vi "dI-dV and Delta.vi"(5 "V offset":dbl, 6 "I offset":dbl, 7 "How many V sweep periods?":dbl=1.0, 8 "Input data":cluster{dbl[], dbl[]}(graph), 9 "dI/dV (Delta) Parameters":T1={"High voltage value"=0.0005, "Low voltage value"=-0.0005, "decimation points"=600, "side points"=4, "polynomial order 2"=3, "valley width"=10, "valley threshold"=1.3e-05, "conductance-peak threshold"=2e-05}) -> (0 "Delta (V)":dbl=7.833333333333333e-05, 1 "Delta":cluster{"2*Delta (V)":dbl, "Delta (V)":dbl}={"2*Delta (V)"=0.00015666666666666666, "Delta (V)"=7.833333333333333e-05} {"2*Delta (V)" format="%#_6p"; "Delta (V)" format="%#_6p"}, 2 "dI/dV and Delta valleys":cluster{"X Subset":dbl[], "Filtered X":dbl[]}[](graph), 3 "I vs V - Offset Plot":cluster{dbl[], dbl[]}[](graph), 4 "Data for second derivative":cluster{"xi used":dbl[], "dX/dt":dbl[]})   [LabVIEW 2016]
uses:
  <vilib>/Analysis/3filter.llb/Savitzky-Golay Filter (DBL).vi
  <vilib>/Analysis/NI_AALPro.lvlib
  <vilib>/gmath/NI_Gmath.lvlib
  <vilib>/Analysis/NI_AALBase.lvlib
  <vilib>/Analysis/NI_AAL_SigProc.lvlib
panel:
  out "High voltage value":dbl=0.0005
  out "Low voltage value":dbl=-0.0005
  out "decimation points":i32=600
  out "side points":i32=4
  out "polynomial order 2":i32=3
  out "valley width":i32=10
  out "valley threshold":dbl=1.3e-05
  out "conductance-peak threshold":dbl=2e-05
  # "paste data here"
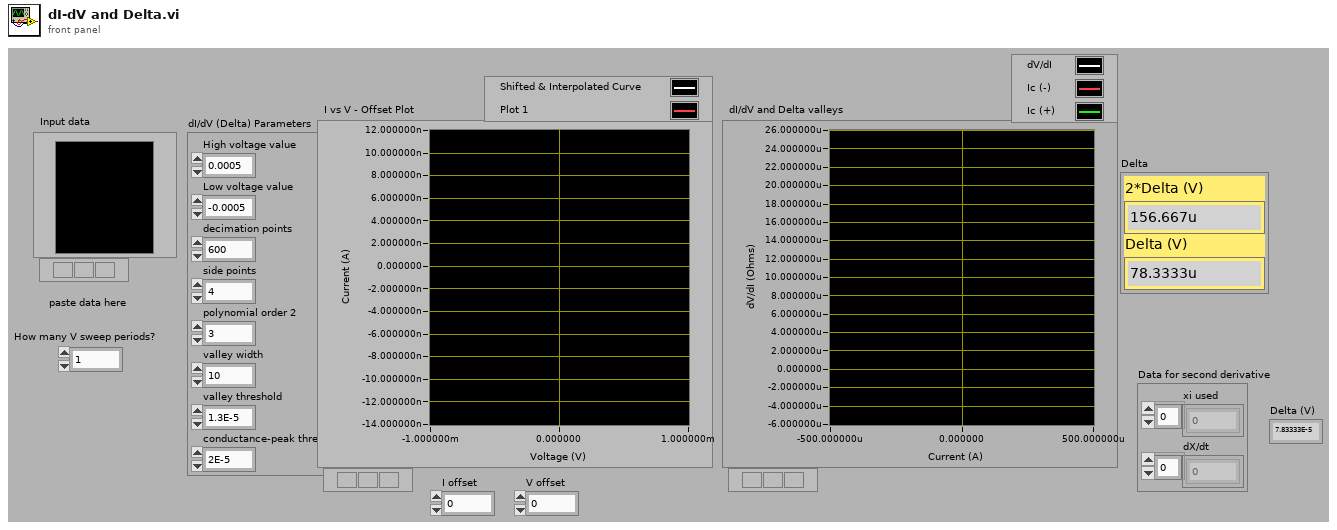
[diagram p1: front panel]
types:
  T1 = cluster{"High voltage value":dbl, "Low voltage value":dbl, "decimation points":i32, "side points":i32, "polynomial order 2":i32, "valley width":i32, "valley threshold":dbl, "conductance-peak threshold":dbl}
  T2 = cluster{"Positive Val":dbl, "Negative Val":dbl, "Ave Ic":dbl}
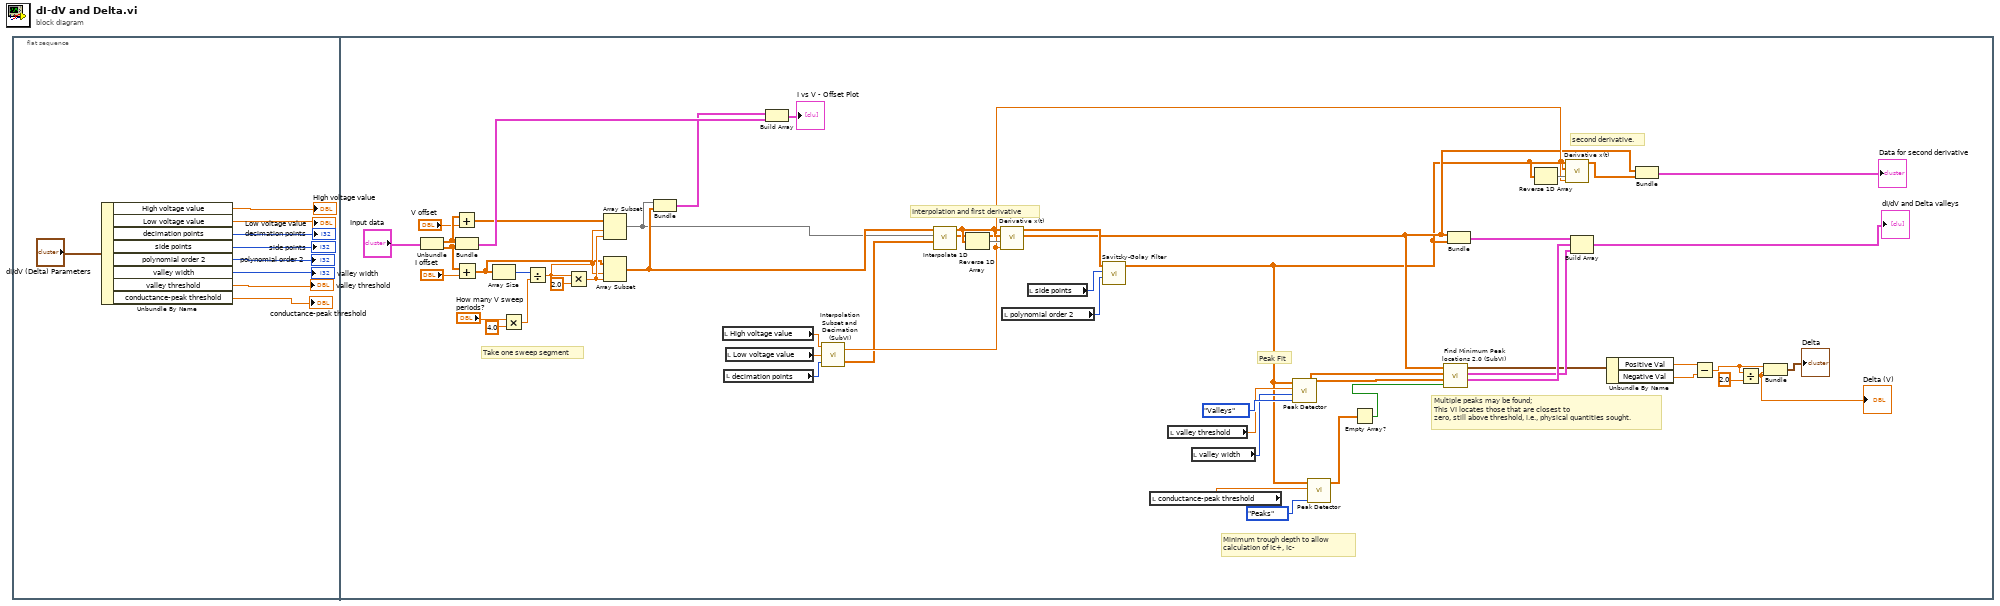
[diagram p0: block diagram]
diagram:
  n1 = flat-sequence {
    frame #0 {
      n2 = Unbundle By Name("dI/dV (Delta) Parameters") -> ("High voltage value"=→"High voltage value":dbl, "Low voltage value"=→"Low voltage value":dbl, "decimation points"=→"decimation points":i32, "side points"=→"side points":i32, "polynomial order 2"=→"polynomial order 2":i32, "valley width"=→"valley width":i32, "valley threshold"=→"valley threshold":dbl, "conductance-peak threshold"=→"conductance-peak threshold":dbl)
    }
    frame #1 {
      # "second derivative."
      # "Multiple peaks may be found;\nThis VI locates those that are closest to\nzero, still above threshold, i.e., physical quantities sought."
      # "Minimum trough depth to allow \ncalculation of Ic+, Ic-"
      # "Peak Fit"
      # "Interpolation and first derivative"
      # "Take one sweep segment"
      n3 = Unbundle("Input data") -> (w61:dbl[], w62:dbl[])
      n4 = Add(x=w61, y="V offset") -> (x+y=w50:dbl[])
      n5 = Bundle(w61, w62) -> (w63:cluster{dbl[], dbl[]})  [unwired: 1 in]
      n6 = Add(x=w62, y="I offset") -> (x+y=w55:dbl[])
      n7 = Array Size(array=w55) -> (size(s)=w51:i32)
      n8 = Multiply(x="How many V sweep periods?", y=4.0) -> (x*y=w52:dbl)
      n9 = Divide(x=w51, y=w52) -> (x/y=w56:dbl)
      n10 = Multiply(x=w56, y=2.0) -> (x*y=w57:dbl)
      n11 = Array Subset(array=w50, index=w56, length=w57) -> (w58:dbl[])
      n12 = Array Subset(array=w55, index=w56, length=w57) -> (w59:dbl[])
      n13 = Bundle(w58, w59) -> (w60:cluster{dbl[], dbl[]})  [unwired: 1 in]
      n14 = local read "High voltage value"() -> (w23:dbl)
      n15 = local read "decimation points"() -> (w21:i32)
      n16 = local read "Low voltage value"() -> (w22:dbl)
      n17 = Build Array(w60, w63) -> (→"I vs V - Offset Plot":cluster{dbl[], dbl[]}[])
      n18 = call "Interpolation Subset and Decimation (SubVI).vi"("decimation points"=w21, "Low value"=w22, "High value"=w23) -> ("Points to use in interpolation (xi)"=w34:dbl[], "Numeric"=w35:dbl)
      n19 = call <vilib>:"Interpolate 1D.vi"("xi"=w34, "X"=w58, "Y"=w59) -> ("xi used"=w29:dbl[], "yi"=w45:dbl[])  [unwired: 6 in, 1 out]
      n20 = Reverse 1D Array(array=w45) -> (reversed array=w46:dbl[])
      n21 = call <vilib>:"Derivative x(t).vi"("dt"=w35, "Final Condition"=w46, "Initial Condition"=w45, "X"=w45) -> ("dX/dt"=w44:dbl[])  [unwired: 6 in, 1 out]
      n22 = local read "polynomial order 2"() -> (w25:i32)
      n23 = local read "side points"() -> (w24:i32)
      n24 = call-poly <vilib>:"Savitzky-Golay Filter.vi"("polynomial order"=w25, "side points"=w24, "X"=w44) -> ("Filtered X"=w19:dbl[])  [unwired: 7 in, 1 out]
      n25 = local read "conductance-peak threshold"() -> (w28:dbl)
      n26 = local read "valley threshold"() -> (w27:dbl)
      n27 = local read "valley width"() -> (w26:i32)
      n28 = call <vilib>:"Peak Detector.vi"("peaks/valleys"=enum32{"Peaks", "Valleys"}."Valleys", "width"=w26, "threshold"=w27, "X"=w19) -> ("Amplitudes"=w37:dbl[], "Locations"=w36:dbl[])  [unwired: 3 in, 3 out]
      n29 = call <vilib>:"Peak Detector.vi"("peaks/valleys"=enum32{"Peaks", "Valleys"}."Peaks", "threshold"=w28, "X"=w19) -> ("Locations"=w42:dbl[])  [unwired: 4 in, 4 out]
      n30 = Empty Array?(array=w42) -> (empty?=w43:bool)
      n31 = call "Find Minimum Peak locations 2.0 (SubVI).vi"("Empty Array?"=w43, "Amplitudes"=w37, "Locations"=w36, "X Array"=w29) -> ("Negative Location"=w39:cluster{dbl[], dbl[]}, "Positive Location"=w38:cluster{dbl[], dbl[]}, "Ic's"=w18:T2)  [unwired: 1 out]
      n32 = Bundle("xi used"=w29, "Filtered X"=w19) -> (w33:cluster{"xi used":dbl[], "Filtered X":dbl[]})  [unwired: 1 in]
      n33 = Reverse 1D Array(array=w19) -> (reversed array=w47:dbl[])
      n34 = call <vilib>:"Derivative x(t).vi"("dt"=w35, "Final Condition"=w47, "Initial Condition"=w19, "X"=w19) -> ("dX/dt"=w48:dbl[])  [unwired: 6 in, 1 out]
      n35 = Build Array(w33, w39, w38) -> (→"dI/dV and Delta valleys":cluster{"xi used":dbl[], "Filtered X":dbl[]}[])
      n36 = Unbundle By Name(w18) -> ("Positive Val"=w17:dbl, "Negative Val"=w16:dbl)
      n37 = Bundle("xi used"=w29, "dX/dt"=w48) -> (→"Data for second derivative":cluster{"xi used":dbl[], "dX/dt":dbl[]})  [unwired: 1 in]
      n38 = Subtract(x=w17, y=w16) -> (x-y=w14:dbl)
      n39 = Divide(x=w14, y=2.0) -> (x/y=w12:dbl)
      "Delta (V)" <- w12
      n40 = Bundle(w14, w12) -> (→"Delta":cluster{dbl, dbl})  [unwired: 1 in]
    }
  }
